vi "Test String To 1D Array.vi"(8 "error in (no error)":errorcluster) -> (0 "error out":errorcluster, 3 "Pass?":bool)   [LabVIEW 2020]
uses:
  G-Unicode/Unicode/Controls/String Encoding.ctl
  G-Unicode/Types/UTF-8 String/UTF-8 String.lvclass/UTF-8 String.ctl
  d266910f-e59a-4c09-865c-c189f5680185.vi
  3294590f-1716-41c0-bf3c-cd8afd0aea86.vi
  99916a31-3c46-4607-a56b-3bfeb49a5e9f.vi
  17bb05e3-0eae-46f4-b435-8620e30f8bbd.vi
  G-Unicode/Unicode/Encode String.vi
  d266910f-e59a-4c09-865c-c189f5680185.vi/46bf550a-28c6-4dfd-813a-9b0ad34779ef.vi
  G-Unicode/Private/Conversion/String as Encoded String.vi
  G-Unicode/Private/Conversion/Polymorphic VIs/String as Encoded String (UTF-8 String).vi
  G-Unicode/Types/UTF-8 String/Write Encoded UTF-8 String.vi
  G-Unicode/Private/Conversion/Polymorphic VIs/String as Encoded String (LabVIEW String).vi
  99916a31-3c46-4607-a56b-3bfeb49a5e9f.vi/46bf550a-28c6-4dfd-813a-9b0ad34779ef.vi
  G-Unicode/Private/Conversion/Text to UTF-8.vi
  G-Unicode/Private/Conversion/Polymorphic VIs/Text to UTF-8 (LabVIEW String).vi
  G-Unicode/Private/Conversion/Encoded UTF-8 String to Encoded UTF-16LE String.vi
  G-Unicode/Unicode/SubVIs/UTF-16 Byte Swap.vi
  G-Unicode/Private/Conversion/UTF-8 to Text.vi
  G-Unicode/Private/Conversion/Polymorphic VIs/UTF-8 to Text (LabVIEW String).vi
  G-Unicode/Private/Conversion/Encoded UTF-16LE String to Encoded UTF-8 String.vi
  G-Unicode/Unicode/Prepend BOM.vi
  G-Unicode/Types/UTF-8 String/Read Encoded UTF-8 String.vi
  G-Unicode/Unicode/SubVIs/Byte Order Marks.vi
  G-Unicode/Unicode/Detect BOM.vi
  G-Unicode/Unicode/Detect String Encoding.vi
  G-Unicode/Types/UTF-8 String/UTF-8 String.lvclass
  G-Unicode/G-Unicode.lvlib
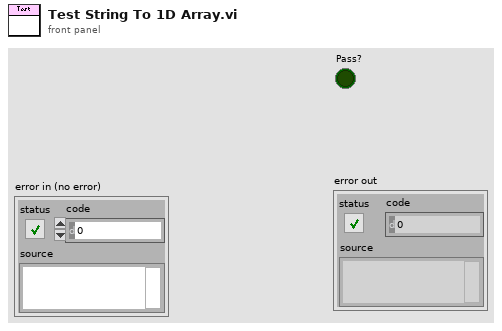
[diagram p1: front panel]
types:
  T1 = typedef "G-Unicode.lvlib/String Encoding.ctl" = enum16{"ANSI", "UTF-8", "UTF-16LE", "UTF-16BE", "Unknown"}
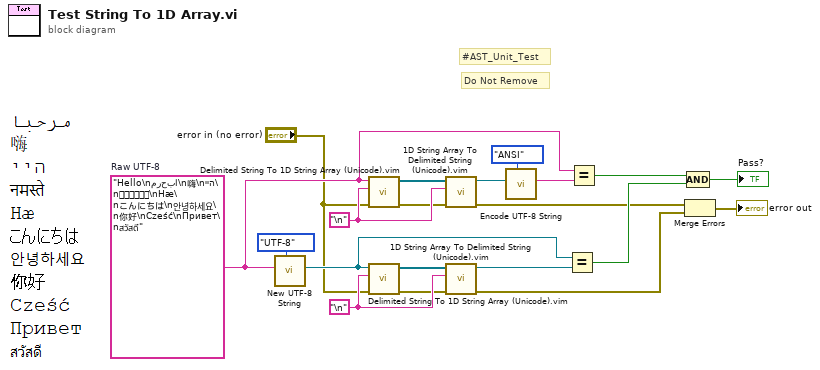
[diagram p0: block diagram]
diagram:
  w16 = "\n"
  w15 = "\n"
  w11 = "Hello\nمرحبا\n嗨\nהיי\nनमस्ते\nHæ\nこんにちは\n안녕하세요\n你好\nCześć\nПривет\nสวัสดี"  # Raw UTF-8
  # "Do Not Remove"
  # "#AST_Unit_Test"
  n1 = call "New UTF-8 String.vi"("Input Encoding (ANSI)"=String_Encoding."UTF-8", "String"=w11) -> ("UTF-8 String"=w10:refnum<class "UTF-8 String.lvclass">)  [unwired: 8 in, 1 out]
  n2 = call "Delimited String To 1D String Array (Unicode).vim"("error in"="error in (no error)", "Delimiter (tab)"=w16, "Delimited String"=w11) -> ("error out"=w6:errorcluster, "String Array"=w17:refnum<class "UTF-8 String.lvclass">[])  [unwired: 7 in]
  n3 = call "Delimited String To 1D String Array (Unicode).vim"("error in"="error in (no error)", "Delimiter (tab)"=w15, "Delimited String"=w10) -> ("error out"=w4:errorcluster, "String Array"=w1:refnum<class "UTF-8 String.lvclass">[])  [unwired: 7 in]
  n4 = call "1D String Array To Delimited String (Unicode).vim"("error in"=w6, "Delimiter (tab)"=w16, "String Array"=w17) -> ("error out"=w2:errorcluster, "Delimited String"=w14:refnum<class "UTF-8 String.lvclass">)  [unwired: 7 in]
  n5 = call "1D String Array To Delimited String (Unicode).vim"("error in"=w4, "Delimiter (tab)"=w15, "String Array"=w1) -> ("error out"=w3:errorcluster, "Delimited String"=w9:refnum<class "UTF-8 String.lvclass">)  [unwired: 7 in]
  n6 = call "Encode UTF-8 String.vi"("Output Encoding (UTF-16LE)"=String_Encoding."ANSI", "UTF-8 String"=w14) -> ("Encoded String"=w12:string)  [unwired: 8 in, 1 out]
  n7 = Equal?(x=w10, y=w9) -> (x = y?=w7:bool)
  n8 = Equal?(x=w11, y=w12) -> (x = y?=w8:bool)
  n9 = Merge Errors(w2, w3) -> (→"error out":errorcluster)
  n10 = Compound Arithmetic op=AND(w8, w7) -> (→"Pass?":bool)
